vi "Event Ctr, Programmable Edge (subVI).vi"(1 "Edge Type (false)":bool, 3 "Reset":bool, 4 "Edge Trigger":bool) -> (0 "16 bit Count":u16)   [LabVIEW 2015]
doc: "This VI supports a hardware selected edge event counter. When the input trigger creates a selected edge, the value of 16-bit Count is incremented on the host VI.\n\nA false value passed to Edge Type will indicate a falling edge count. A true value passed to Edge Type will indicate a rising edge count."
panel:
  # "This VI supports a hardware selected edge event counter.  When the input trigger creates a selected edge, the value of 16-bit Count is incremented on the host VI.\n\nA false value passed to Edge Type will indicate a falling edge count.  A true value passed to Edge Type will indicate a rising edge count."
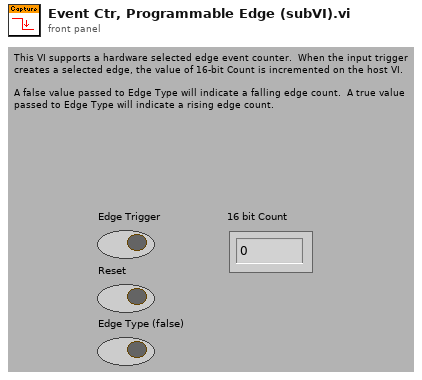
[diagram p1: front panel]
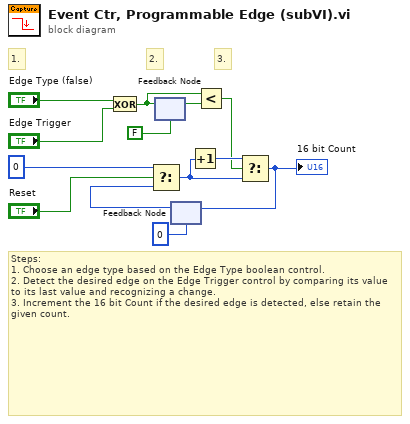
[diagram p0: block diagram]
diagram:
  # "3."
  # "2."
  # "1."
  # "Steps:\n1. Choose an edge type based on the Edge Type boolean control.\n2. Detect the desired edge on the Edge Trigger control by comparing its value to its last value and recognizing a change.\n3. Increment the 16 bit Count if the desired edge is detected, else retain the given count."
  n1 = Exclusive Or(1:"Edge Trigger", 2:"Edge Type (false)") -> (0:w6:bool)
  n2 = feedback-in #1(w6) -> ()
  n3 = feedback #1(FALSE) -> (w5:bool)
  n4 = feedback #2(u16 0 ("16 bit")) -> (w4:u16)
  n5 = Select(t=u16 0 ("16 bit"), s="Reset", f=w4) -> (s? t:f=w10:u16)
  n6 = Increment(x=w10) -> (x+1=w9:u16)
  n7 = Less?(x=w6, y=w5) -> (x < y?=w8:bool)
  n8 = Select(t=w9, s=w8, f=w10) -> (s? t:f=w3:u16)
  "16 bit Count" <- w3
  n9 = feedback-in #2(w3) -> ()
